vi "lab2_3 (1).vi"() -> ()   [LabVIEW 2025]
uses:
  <vilib>/Analysis/2dsp.llb/Real FFT.vi
  <vilib>/measure/NI_MABase.lvlib
  <vilib>/Analysis/NI_AALPro.lvlib
panel:
  out "Waveform Graph 2":dbl[](graph)
  out "Waveform Graph":waveform(dbl)(graph)
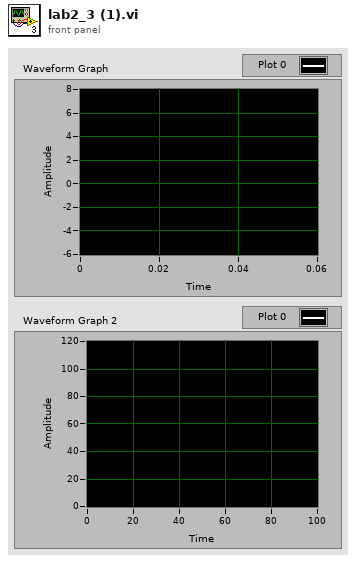
[diagram p1: front panel]
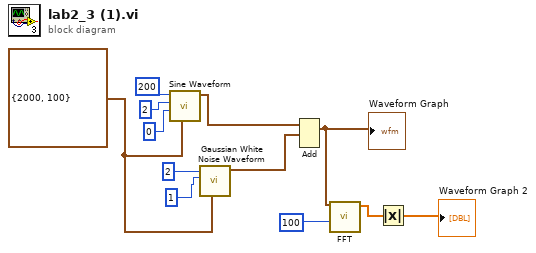
[diagram p0: block diagram]
diagram:
  w10 = cluster{i32, i32} {2000, 100}
  n1 = call <vilib>:"Sine Waveform.vi"("sampling info"=w10, "phase"=0, "amplitude"=2, "frequency"=200) -> ("signal out"=w6:waveform(dbl))  [unwired: 6 in, 1 out]
  n2 = call <vilib>:"Gaussian White Noise Waveform.vi"("sampling info"=w10, "seed"=1, "standard deviation"=2) -> ("signal out"=w5:waveform(dbl))  [unwired: 7 in, 1 out]
  n3 = Add(1:w5, 2:w6) -> (0:w2:waveform(dbl))  [unwired: 1 in, 1 out]
  "Waveform Graph" <- w2
  n4 = call-poly <vilib>:"FFT.vi"("FFT size"=100, "X"=w2) -> ("FFT {X}"=w4:cdb[])  [unwired: 8 in, 1 out]
  n5 = Absolute Value(x=w4) -> (abs(x)=→"Waveform Graph 2":dbl[])
